vi "Get Module Configuration.vi"(8 "error in (no error)":errorcluster, 11 "Data Cluster":T1) -> (0 "error out":errorcluster, 2 "Configuration":T2, 3 "Data Cluster dup":T1)   [LabVIEW 2014, in "Configurable.lvlib"]
uses:
  Configurable.lvlib
  ModuleConfiguration--Cluster.ctl
  Module Data--cluster.ctl
  <vilib>/LabVIEW Open Source/Configuration Manager/Manager/ConfigManager.lvclass
  <vilib>/LabVIEW Open Source Project/Unicity/UniqueName/UniqueNameClass/UniqueName.lvclass
  <vilib>/LabVIEW Open Source Project/Unicity/UniqueName/UniqueNameClass/UniqueName.lvclass/UniqueName.ctl
  <vilib>/LabVIEW Open Source/Configuration Manager/Manager/ConfigManager.lvclass/ConfigManager.ctl
  <vilib>/LabVIEW Open Source/Configuration Manager/Manager/Read.vi
  <vilib>/LabVIEW Open Source/Configuration Manager/Manager/Read Serializer.vi
  <vilib>/LabVIEW Open Source/Configuration Manager/Manager/Read Encoding.vi
  <vilib>/LabVIEW Open Source/Configuration Manager/Manager/Read Encryption.vi
  <vilib>/LabVIEW Open Source/Configuration Manager/Manager/Write.vi
  <vilib>/LabVIEW Open Source/Configuration Manager/Manager/Decompose KVPs.vi
  <vilib>/Utility/VariantDataType/GetTypeInfo.vi
  <vilib>/LabVIEW Open Source/Data Manipulation/KVP Parser.vi
  <vilib>/LabVIEW Open Source/Configuration Manager/Cache/ConfigManager.Cache.lvclass
  <vilib>/LabVIEW Open Source/Configuration Manager/Encoding/Encoding.lvclass
  <vilib>/LabVIEW Open Source/Configuration Manager/Encryption/Encryption.lvclass
  <vilib>/LabVIEW Open Source/Configuration Manager/Serializer/Serializer.lvclass
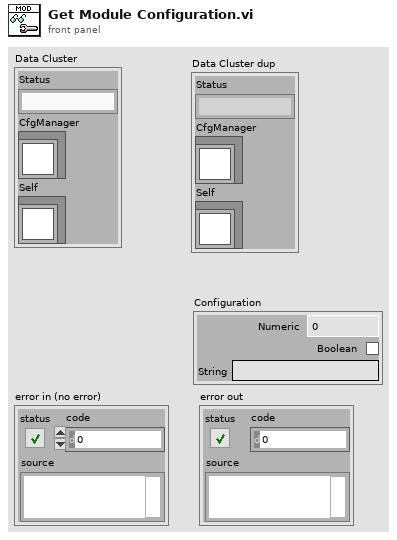
[diagram p1: front panel]
types:
  T1 = typedef "Configurable.lvlib/Module Data--cluster.ctl" = cluster{"Status":string, "CfgManager":refnum<class "ConfigManager.lvclass">, "Self":refnum<class "UniqueName.lvclass">}
  T2 = typedef "Configurable.lvlib/ModuleConfiguration--Cluster.ctl" = cluster{"Numeric":dbl, "Boolean":bool, "String":string}
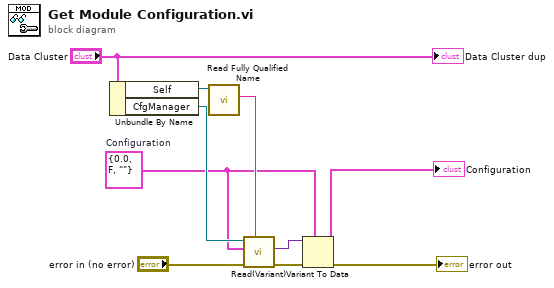
[diagram p0: block diagram]
diagram:
  w2 = T2 {"Numeric"=0.0, "Boolean"=FALSE, "String"=""}  # Configuration
  n1 = Unbundle By Name("Data Cluster") -> ("Self"=w4:refnum<class "UniqueName.lvclass">, "CfgManager"=w5:refnum<class "ConfigManager.lvclass">)
  n2 = call <vilib>:"Read Fully Qualified Name.vi"("UniqueName in"=w4) -> ("Fully Qualified Name"=w6:string)  [unwired: 9 in, 1 out]
  n3 = call <vilib>:"Read(Variant).vi"("Qualified Name"=w6, "error in (no error)"="error in (no error)", "Type"=w2, "ConfigManager in"=w5) -> ("error out"=w8:errorcluster, "value"=w7:variant)  [unwired: 3 in, 3 out]
  n4 = Variant To Data(error in=w8, type=w2, Variant=w7) -> (data=→"Configuration":T2, error out=→"error out":errorcluster)
  "Data Cluster dup" <- "Data Cluster"
